vi "Find_Source_Item_By_Path.vi"(8 "error in (no error)":errorcluster, 10 "Path":path, 11 "AB_Build.lvclass":refnum<class "AB_Build.lvclass">) -> (0 "error out":errorcluster, 3 "Found Source Item":refnum<class "AB_Source.lvclass">)   [LabVIEW 2020, in "AB_Build.lvclass"]
uses:
  <vilib>/AppBuilder/AB_Classes/Build/AB_Build.lvclass
  <vilib>/AppBuilder/AB_Classes/Source/AB_Source.lvclass
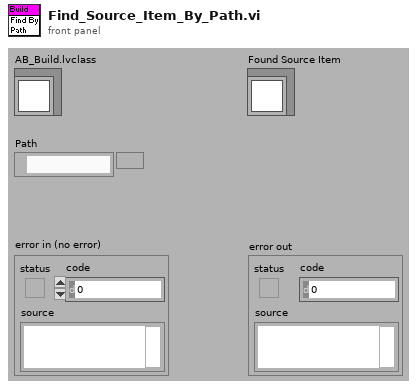
[diagram p1: front panel]
types:
  T1 = typedef "AB_Source.ctl" = cluster{"path":path, "itemID":string, "parentIndex":i32, "sourceInclusion":T2, "destinationIndex":i32, "properties":T3[], "newName":string, "lvfile":bool, "valid":bool, "eng_inBuild":bool, "eng_isNonVILink":bool, "Amalgamation":bool, "Amalgamation Piece":bool, "eng_delimitedName":string, "preventRename":bool}
  T2 = typedef "AB_Source_Inclusion.ctl" = enum16{"IncludeIfReferenced", "Include", "Exclude", "TopLevel"}
  T3 = typedef "AB_Source_Properties.ctl" = cluster{"sourcePropertyType":T4, "value":variant}
  T4 = typedef "AB_Source_Property_Type.ctl" = enum16{"Remove block diagram", "Remove front panel", "Password", "Window has title bar", "Show menu bar", "Show vertical scroll bar", "Show horizontal scroll bar", "Show toolbar", "Show Abort button", "Show fp when called", "Window behavior", "Allow user to close window", "Window run-time position", "Run when opened", "Allow debugging", "Auto error handling", "Generate guard code", "Use stack variables", "Expression folding", "Integer only", "Inline subVI"}
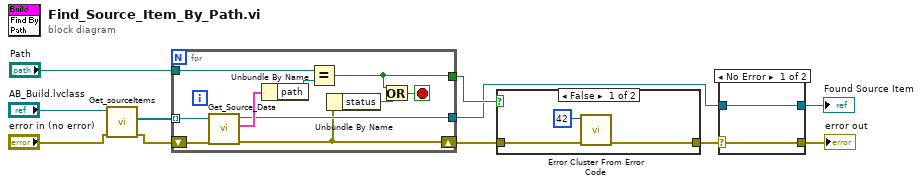
[diagram p0: block diagram]
diagram:
  n1 = call <vilib>:"Get_sourceItems.vi"("error in (no error)"="error in (no error)", "Class in"="AB_Build.lvclass") -> ("error out"=w9:errorcluster, "sourceItems"=w7:refnum<class "AB_Source.lvclass">[])  [unwired: 8 out]
  n2 = for {
    tunnel: "Path" -> [w19]
    tunnel: w7 -> [w21] mode=indexing
    tunnel: [w18] -> w3
    tunnel: [w16] -> w10
    shift-right: [w15] -> w11
    shift-left: w9 -> [w17]
    stop <- w14 stop-if-true
    n3 = call <vilib>:"Get_Source_Data.vi"("error in (no error)"=w17, "Class in"=w21) -> ("error out"=w15:errorcluster, "data"=w20:T1, "Class out"=w18:refnum<class "AB_Source.lvclass">)  [unwired: 7 out]
    n4 = Unbundle By Name(w20) -> ("path"=w12:path)
    n5 = Equal?(x=w19, y=w12) -> (x = y?=w16:bool)
    n6 = Unbundle By Name(w15) -> ("status"=w13:bool)
    n7 = Or(x=w16, y=w13) -> (x .or. y?=w14:bool)
  }
  n8 = case shown="False" w10 {
    tunnel: w11 -> [w23 w25]
    tunnel: [w22 w25] -> w4
    frame False {
      n9 = call <vilib>:"Error Cluster From Error Code.vi"("error in (no error)"=w23, "error code (0)"=42) -> ("error out"=w22:errorcluster)  [unwired: 1 in, 6 out]
    }
    frame True {
    }
  }
  n10 = case shown="No Error" w4 {
    selector: w4 -> [w26 w28]
    tunnel: w3 -> [w27 _]
    tunnel: [w27 _] -> w2
    tunnel: [w26 w28] -> w1
    frame No Error {
    }
    frame Error {
    }
  }
  "error out" <- w1
  "Found Source Item" <- w2
